vi "Handle Error.vi"(8 "error in (no error)":errorcluster, 11 "Auto UI in":refnum<class "Auto UI.lvclass">) -> (0 "error out":errorcluster, 2 "stop actor?":bool=TRUE, 3 "Auto UI out":refnum<class "Auto UI.lvclass">)   [LabVIEW 2023, in "GUI.lvlib" / "Auto UI.lvlib" / "Auto UI.lvclass"]
doc: "(<B>Filename</B>: Actor Framework.lvlib:Actor.lvclass:Handle Error.vi)\n\nDefines how the actor handles an error that occurred while processing a message. By default, this method does nothing except stop the actor."
uses:
  Auto UI.lvclass
  Reused Code/Subpanels Actor/subpanels/subpanel/subpanel (abstract).lvclass
  GUI.lvlib
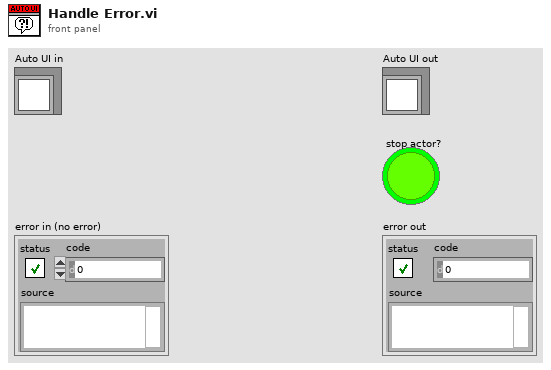
[diagram p1: front panel]
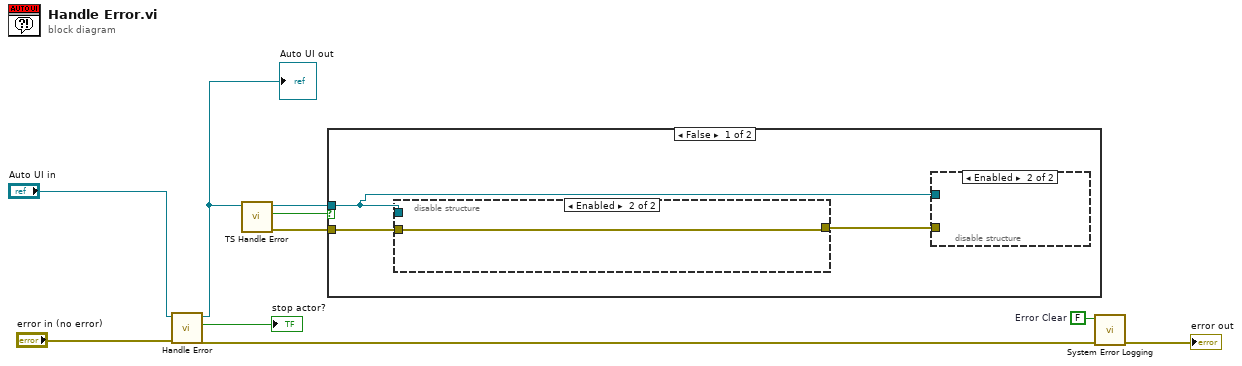
[diagram p0: block diagram]
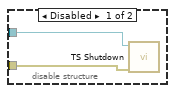
[diagram p2: hidden frame]
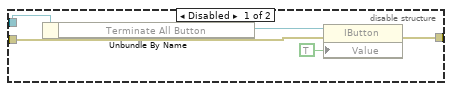
[diagram p3: hidden frame]
diagram:
  w2 = FALSE  # Error Clear
  n1 = call-parent "Handle Error.vi"("error in (no error)"="error in (no error)", "Actor in"="Auto UI in") -> ("error out"=w4:errorcluster, "stop actor?"=→"stop actor?":bool, "Actor out"=w7:refnum<class "Auto UI.lvclass">)  [unwired: 7 in]
  "Auto UI out" <- w7
  n2 = call "TS Handle Error.vi"("Auto UI in"=w7) -> ("error out"=w1:errorcluster, "IsStarted"=w6:bool, "Auto UI out"=w5:refnum<class "Auto UI.lvclass">)  [unwired: 8 in]
  n3 = case shown="False" w6 {
    tunnel: w5 -> [w11 _]
    tunnel: w1 -> [w13 _]
    frame False {
      n4 = disable-structure shown="Enabled" {
        disable-tunnel: w13 -> [w18 w21]
        disable-tunnel: [w17 w21] -> w12
        disable-tunnel: w11 -> [w16 _]
        frame Disabled {
          n5 = Unbundle By Name(w16) -> ("Terminate All Button"=w20:refnum<k7>)
          n6 = property class="IButton"(reference=w20, error in=w18, "Value"=TRUE) -> (error out=w17:errorcluster)  [unwired: 1 out]
        }
        frame Enabled {
        }
      }
      n7 = disable-structure shown="Enabled" {
        disable-tunnel: w12 -> [w15 _]
        disable-tunnel: w11 -> [w14 _]
        frame Disabled {
          n8 = call "TS Shutdown.vi"("error in (no error)"=w15, "Auto UI in"=w14) -> ()  [unwired: 8 in, 2 out]
        }
        frame Enabled {
        }
      }
    }
    frame True {
    }
  }
  n9 = call "System Error Logging.vi"("error in"=w4, "Error Clear"=w2) -> ("error out"=→"error out":errorcluster)  [unwired: 9 in]
